vi "Discrete State-Space.vi"(0 "input points":dbl[](array[numeric]) format="%.2f", 1 "initial conditions":dbl[](array[numeric]) format="%.2f", 3 "MIMO state space":T1 {"D" format="%.2f"; "C" format="%.2f"; "B" format="%.2f"; "A" format="%.2f"}, 4 "initialize":bool) -> (5 "output points":dbl[](array[numeric]) format="%.2f", 6 "states":dbl[](array[numeric]) format="%.2f")   [LabVIEW 2020, in "NI_AdvCtrl_discrete linear.lvlib"]
doc: "LabVIEW no longer supports this VI. You can obtain similar functionality by installing the LabVIEW Simulation Module.\n\nCalculates a set of new output points where the system description, the input points, and the initial conditions are given. The system description is based on x[n+1]=Ax[n]+Bu[n] and y[n]=Cx[n]+Du[n]."
uses:
  <vilib>/addons/control/advanced/NI_AdvCtrl_discrete linear.lvlib
  <vilib>/addons/control/advanced/NI_AdvCtrl_continuous linear.lvlib
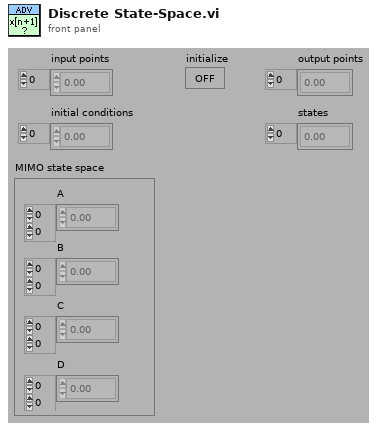
[diagram p1: front panel]
types:
  T1 = cluster{"A":dbl[][], "B":dbl[][], "C":dbl[][], "D":dbl[][]}
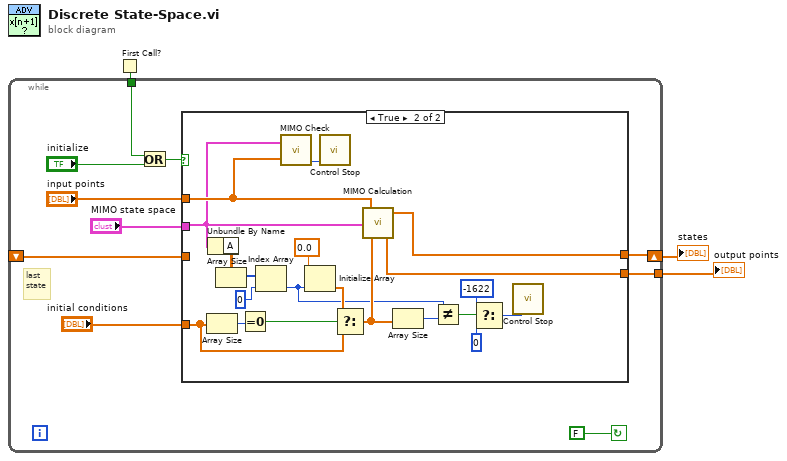
[diagram p0: block diagram]
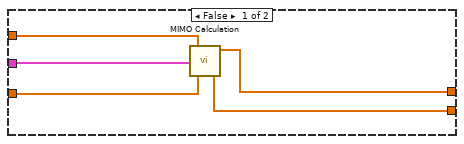
[diagram p2: hidden frame]
diagram:
  n1 = First Call?() -> (First Call?: T/F=w1:bool)
  n2 = while {
    tunnel: w1 -> [w8]
    tunnel: [w12] -> w3
    shift-left: _ -> [w13]
    shift-right: [w11] -> w2
    stop <- FALSE continue-if-true
    # "last\nstate"
    n3 = Or(x=w8, y="initialize") -> (x .or. y?=w7:bool)
    n4 = case shown="True" w7 {
      tunnel: [w17 w38] -> w12
      tunnel: "MIMO state space" -> [w18 w22]
      tunnel: "input points" -> [w16 w23]
      tunnel: w13 -> [w15 _]
      tunnel: [w14 w37] -> w11
      tunnel: "initial conditions" -> [_ w32]
      frame False {
        n5 = call <vilib>:"MIMO Calculation.vi"("x(n)"=w15, "MIMO State-Space"=w18, "u(n)"=w16) -> ("y(n)"=w17:dbl[], "x(n+1)"=w14:dbl[])
      }
      frame True {
        n6 = Array Size(array=w32) -> (size(s)=w35:i32)
        n7 = Unbundle By Name(w22) -> ("A"=w21:dbl[][])
        n8 = Array Size(array=w21) -> (size(s)=w29:i32[])
        n9 = Equal To 0?(x=w35) -> (x = 0?=w33:bool)
        n10 = Index Array(array=w29, index=0 ("Index")) -> (element=w20:i32)
        n11 = call <vilib>:"MIMO Check.vi"("MIMO State-Space"=w22, "Input Points"=w23) -> ("error"=w36:i32)  [unwired: 3 out]
        n12 = Initialize Array(0.0, w20) -> (w31:dbl[])
        n13 = call <vilib>:"Control Stop.vi"("error"=w36) -> ()  [unwired: 2 out]
        n14 = Select(t=w31, s=w33, f=w32) -> (s? t:f=w30:dbl[])
        n15 = call <vilib>:"MIMO Calculation.vi"("x(n)"=w30, "MIMO State-Space"=w22, "u(n)"=w23) -> ("y(n)"=w38:dbl[], "x(n+1)"=w37:dbl[])
        n16 = Array Size(array=w30) -> (size(s)=w28:i32)
        n17 = Not Equal?(x=w20, y=w28) -> (x != y?=w27:bool)
        n18 = Select(t=-1622, s=w27, f=0) -> (s? t:f=w26:i32)
        n19 = call <vilib>:"Control Stop.vi"("error"=w26) -> ()  [unwired: 2 out]
      }
    }
  }
  "output points" <- w3
  "states" <- w2
